vi "Update Waveform.vi"(8 "error in (no error)":errorcluster, 11 "Sine in":refnum<class "Sine.lvclass">) -> (0 "error out":errorcluster, 3 "Sine out":refnum<class "Sine.lvclass">)   [LabVIEW 2016, in "Sine.lvclass"]
uses:
  Sine.lvclass
  C:/Users/fflores/Documents/LabVIEW-Open-Projects/Signal Generator OOP/Waveform/Waveform.lvclass
  Waveform/Waveform.lvclass/Waveform.ctl
  Waveform/Waveform.lvclass
  <vilib>/measure/NI_MABase.lvlib
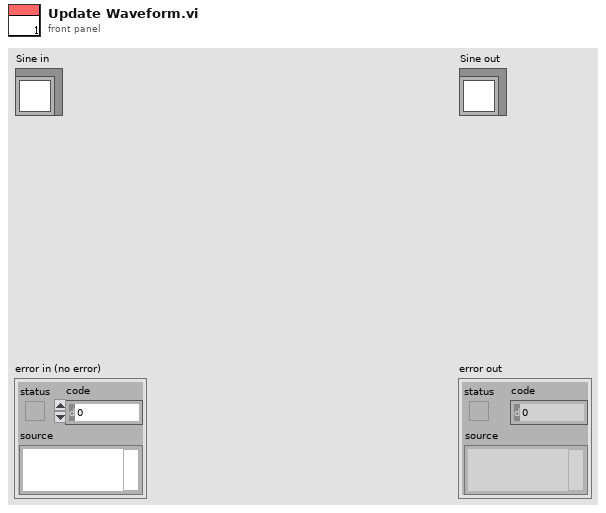
[diagram p1: front panel]
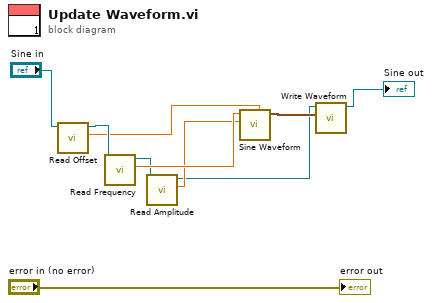
[diagram p0: block diagram]
diagram:
  n1 = call "Read Offset.vi"("Waveform in"="Sine in") -> ("Offset"=w7:dbl, "Waveform out"=w8:refnum<class "Sine.lvclass">)  [unwired: 8 in, 1 out]
  n2 = call "Read Frequency.vi"("Waveform in"=w8) -> ("Frequency"=w6:dbl, "Waveform out"=w4:refnum<class "Sine.lvclass">)  [unwired: 8 in, 1 out]
  n3 = call "Read Amplitude.vi"("Waveform in"=w4) -> ("Amplitude"=w5:dbl, "Waveform out"=w3:refnum<class "Sine.lvclass">)  [unwired: 8 in, 1 out]
  n4 = call <vilib>:"Sine Waveform.vi"("offset"=w7, "amplitude"=w5, "frequency"=w6) -> ("signal out"=w9:waveform(dbl))  [unwired: 7 in, 1 out]
  n5 = call "Write Waveform.vi"("Waveform"=w9, "Waveform in"=w3) -> ("Waveform out"=→"Sine out":refnum<class "Sine.lvclass">)  [unwired: 8 in, 1 out]
  "error out" <- "error in (no error)"
